vi "test.vi"() -> ()   [LabVIEW 2009]
uses:
  Camera.lvlib
  Lens Distortion.lvlib
  ImageProcessing.lvlib
panel:
  out "Em 2":T1(plugin-control)
  out "Corr":T1(plugin-control)
  out "Em":T1(plugin-control)
  out "Calib":T1(plugin-control)
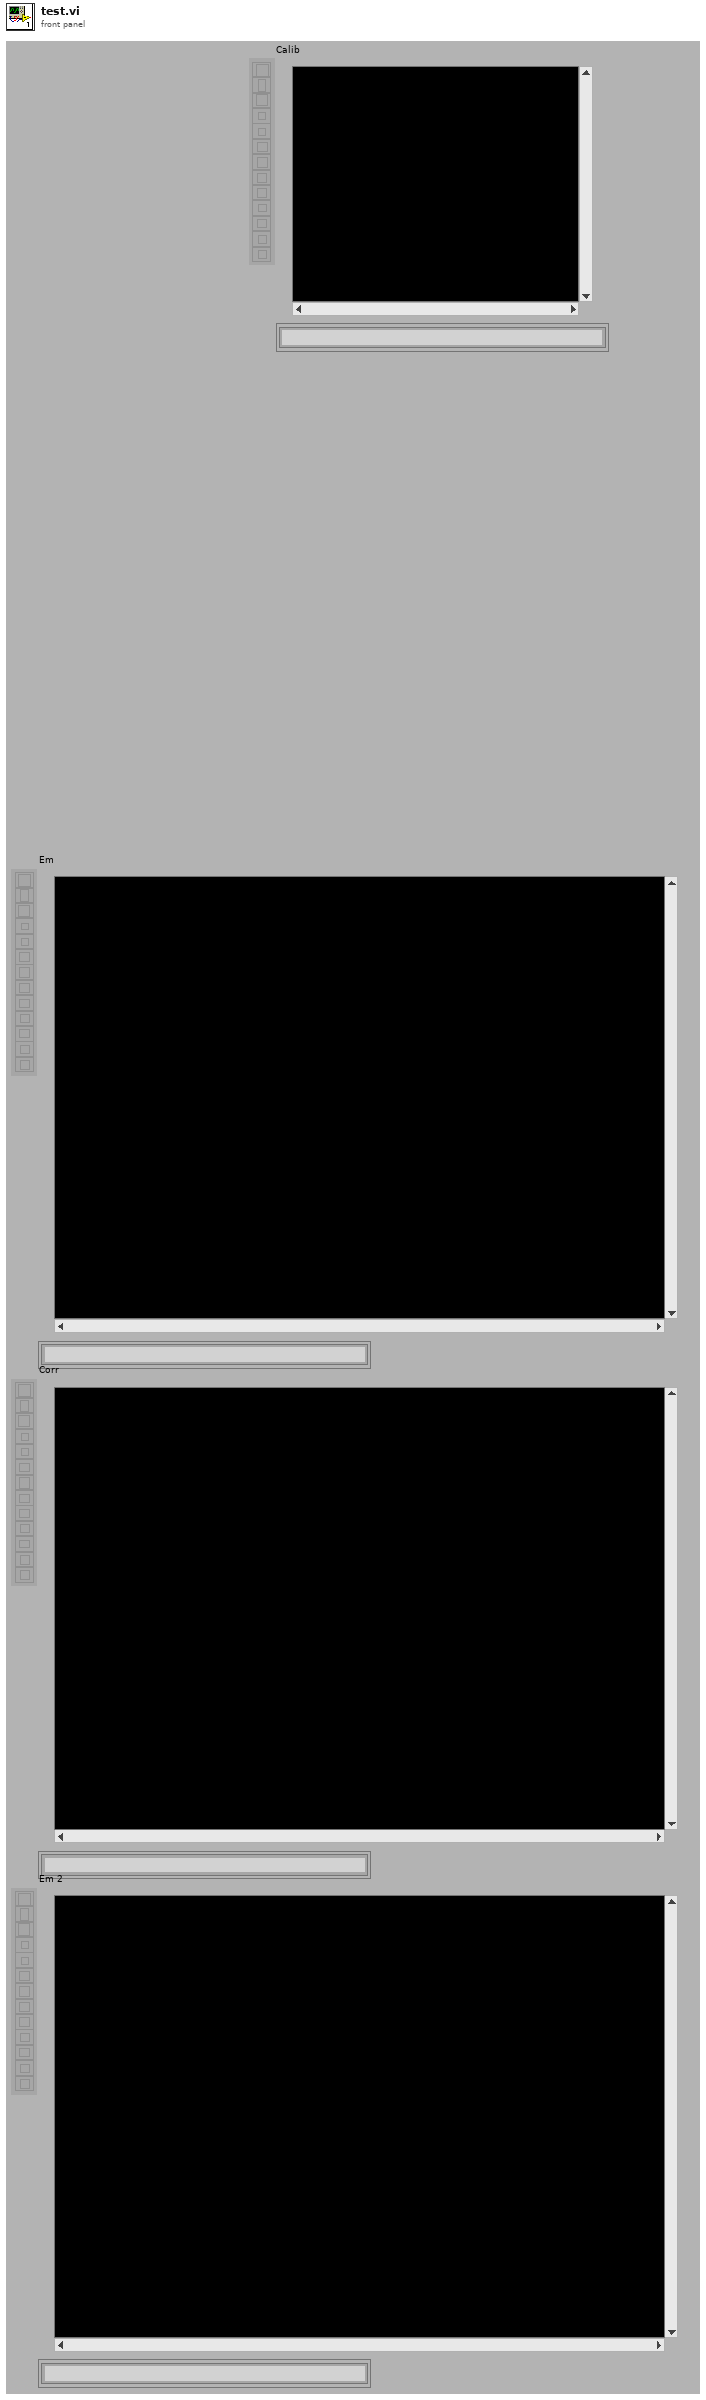
[diagram p1: front panel]
types:
  T1 = typedef "IMAQ Image.ctl" = refnum<image>
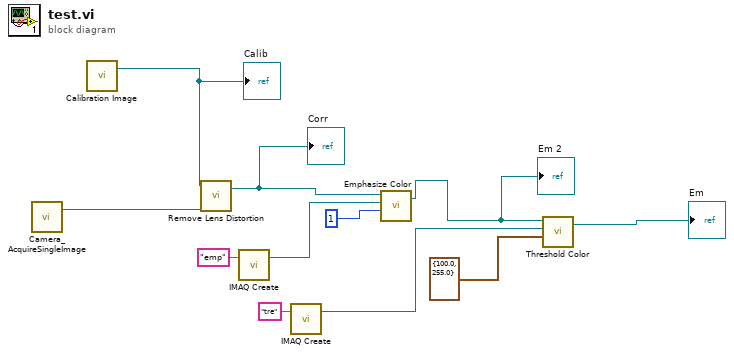
[diagram p0: block diagram]
diagram:
  n1 = call "Camera_AcquireSingleImage.vi"() -> ("Image Out"=w10:T1)  [unwired: 2 in, 1 out]
  n2 = call "Calibration Image.vi"() -> ("Calibration Image"=w11:T1)  [unwired: 2 in, 1 out]
  "Calib" <- w11
  n3 = call "Remove Lens Distortion.vi"("Image Dst"=w10, "Calibration Image"=w11) -> ("Corrected Image"=w2:T1)  [unwired: 1 in, 1 out]
  "Corr" <- w2
  n4 = call "IMAQ Create"("Image Name"="emp") -> ("New Image"=w6:T1)  [unwired: 4 in, 1 out]
  n5 = call "IMAQ Create"("Image Name"="tre") -> ("New Image"=w3:T1)  [unwired: 4 in, 1 out]
  n6 = call "Emphasize Color.vi"("Color"=i8 1, "Image Dst"=w6, "Image Src"=w2) -> ("Image Out"=w1:T1)  [unwired: 1 in, 1 out]
  "Em 2" <- w1
  n7 = call "Threshold Color.vi"("Range"=cluster{"Lower value":sgl, "Upper value":sgl} {"Lower value"=100.0, "Upper value"=255.0}, "Image Dst"=w3, "Image Src"=w1) -> ("Image Dst Out"=→"Em":T1)  [unwired: 1 in, 1 out]
